vi "MMC_sendCommand.vi"(2 "Error in":errorcluster, 3 "Command String":string) -> (0 "Error out":errorcluster, 1 "function return":i32)   [LabVIEW 2024]
doc: "This vi sends a command string"
uses:
  MMC.dll
panel:
  # "MMC_sendCommand"
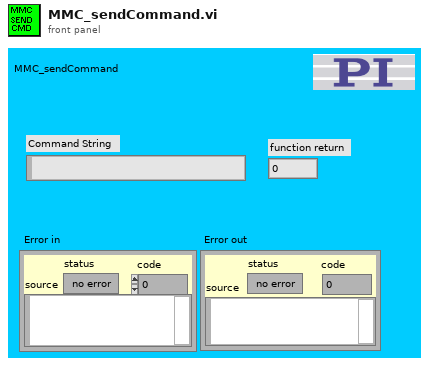
[diagram p1: front panel]
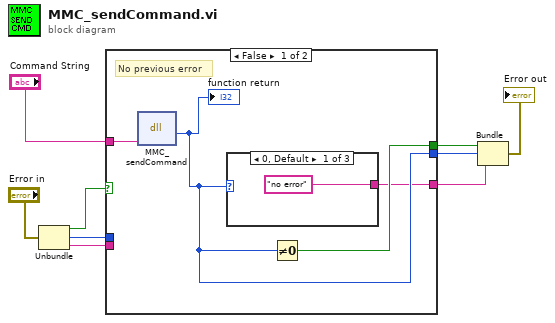
[diagram p0: block diagram]
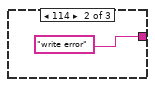
[diagram p2: hidden frame]
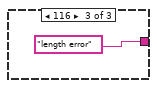
[diagram p3: hidden frame]
diagram:
  n1 = Unbundle("Error in") -> ("status"=w3:bool, "code"=w1:i32, "source"=w2:string)
  n2 = case shown="False" w3 {
    selector: w3 -> [_ w17]
    tunnel: [w13 w18] -> w9
    tunnel: "Command String" -> [w12 _]
    tunnel: [w11 w17] -> w7
    tunnel: [w10 w19] -> w5
    tunnel: w2 -> [_ w19]
    tunnel: w1 -> [_ w18]
    frame False {
      # "No previous error"
      n3 = dll-call lib="E:/Wilson/HoppingSICM_TK/HoppingSICM_v1/DLLs/MMC.dll" fn="MMC_sendCommand"("command"=w12) -> (w13:i32)  [unwired: 4 in, 2 out]
      "function return" <- w13
      n4 = case shown="0, Default" w13 {
        tunnel: ["no error" "write error" "length error"] -> w10
        frame 0, Default {
        }
        frame 114 {
        }
        frame 116 {
        }
      }
      n5 = Not Equal To 0?(x=w13) -> (x != 0?=w11:bool)
    }
    frame True {
      # "error in"
    }
  }
  n6 = Bundle(w7, "code"=w9, "source"=w5) -> (→"Error out":cluster{bool, "code":i32, "source":string})  [unwired: 1 in]
